vi "Get Session ID.vi"(11 "IWelcomeHandler in":refnum<class "IWelcomeHandler.lvclass">) -> (2 "Session ID":u64, 3 "IWelcomeHandler out":refnum<class "IWelcomeHandler.lvclass">)   [LabVIEW 2020, in "wamplv.lvlib" / "IWelcomeHandler.lvclass"]
uses:
  IWelcomeHandler.lvclass
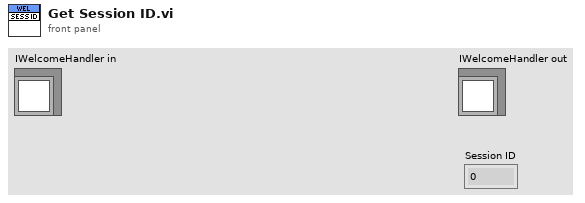
[diagram p1: front panel]
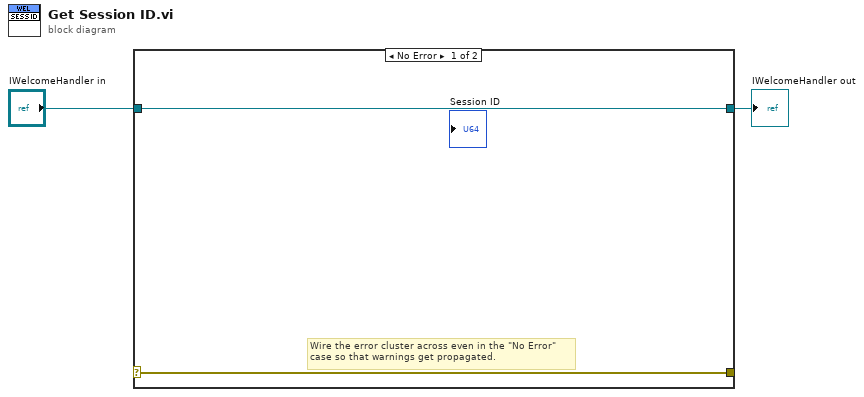
[diagram p0: block diagram]
diagram:
  n1 = case shown="No Error" w4 {
    selector: [w5 w8] -> w4
    tunnel: [w5 w8] -> w3
    tunnel: [w6 w7] -> w1
    tunnel: "IWelcomeHandler in" -> [w6 w7]
    frame No Error {
      # "Wire the error cluster across even in the \"No Error\"\ncase so that warnings get propagated."
    }
    frame Error {
    }
  }
  "IWelcomeHandler out" <- w1
